vi "Target Gallon Fill Time.vi"(7 "Target Gallons":dbl, 8 "Error In":errorcluster, 9 "GEA Inputs":T1 {"Destination" format="%.0x"; "Source" format="%.0x"}, 10 "Standalone?":bool, 11 "GEA2 Reference In":refnum<k24>) -> (0 "Error Out":errorcluster, 2 "Target Gallon Fill Time (sec)":dbl, 3 "GEA2 Reference Out":refnum<k24>)   [LabVIEW 2016, in "TLMB.lvlib"]
uses:
  Projects/TLMB.lvlib
  Q:/Common/DLLs/GEA3/GeaCommunication.dll
  Common/DLLs/GEA3/GeaCommunication.dll
  Common/LabVIEW GEA2 Toolkit/LabVIEW_GEA2_Toolkit.lvlibp/type defs/Source_Destination.ctl
  Common/LabVIEW GEA2 Toolkit/LabVIEW_GEA2_Toolkit.lvlibp/type defs/ERD Read Data In.ctl
  Common/LabVIEW GEA2 Toolkit/LabVIEW_GEA2_Toolkit.lvlibp/type defs/Data Type.ctl
  Common/LabVIEW GEA2 Toolkit/LabVIEW_GEA2_Toolkit.lvlibp
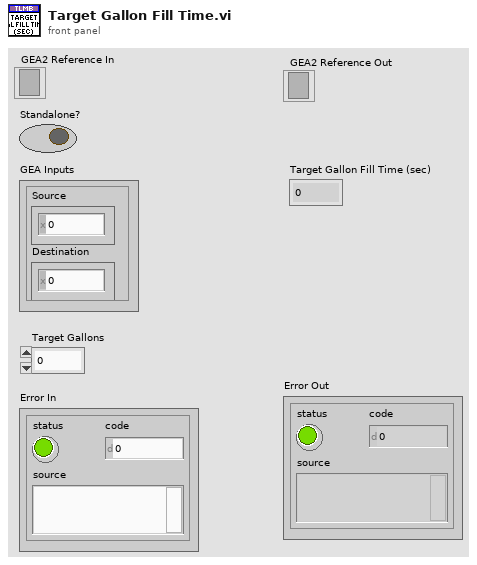
[diagram p1: front panel]
types:
  T1 = typedef "LabVIEW_GEA2_Toolkit.lvlibp/Source_Destination.ctl" = cluster{"Source":u8, "Destination":u8}
  T2 = typedef "LabVIEW_GEA2_Toolkit.lvlibp/ERD Read Data In.ctl" = cluster{"ERD Number":u16, "Data Type":T3}
  T3 = typedef "LabVIEW_GEA2_Toolkit.lvlibp/Data Type.ctl" = enum16{"string", "boolean", "uint8_t", "uint16_t", "uint32_t", "uint64_t", "int8_t", "int16_t", "int32_t", "int64_t"}
  T4 = typedef "LabVIEW_GEA2_Toolkit.lvlibp/ERD Read Data Out.ctl" = cluster{"ERD Number":u16, "Data":string}
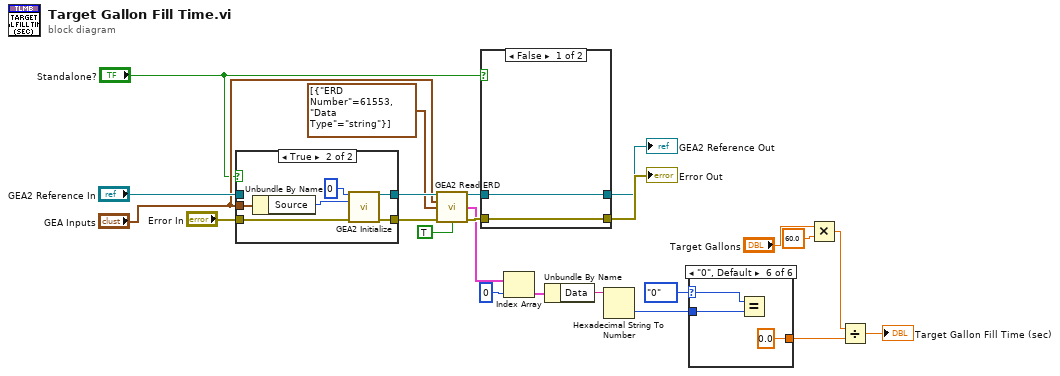
[diagram p0: block diagram]
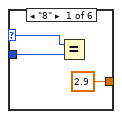
[diagram p2: hidden frame]
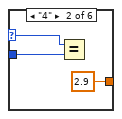
[diagram p3: hidden frame]
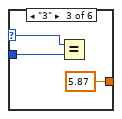
[diagram p4: hidden frame]
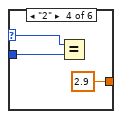
[diagram p5: hidden frame]
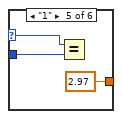
[diagram p6: hidden frame]
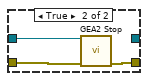
[diagram p7: hidden frame]
diagram:
  n1 = case shown="True" "Standalone?" {
    tunnel: "Error In" -> [w24 w31]
    tunnel: [w24 w30] -> w23
    tunnel: "GEA2 Reference In" -> [w25 _]
    tunnel: [w25 w29] -> w18
    tunnel: "GEA Inputs" -> [_ w27]
    frame False {
    }
    frame True {
      n2 = Unbundle By Name(w27) -> ("Source"=w28:u8)
      n3 = call "GEA2 Initialize.vi"("Board Index"=0, "Source Address"=w28, "error in"=w31) -> ("GEA2 Reference Out"=w29:refnum<k24>, "error out"=w30:errorcluster)  [unwired: 10 in, 1 out]
    }
  }
  n4 = call "GEA2 Read ERD.vi"("GEA2 Reference In"=w18, "GEA Inputs"="GEA Inputs", "Read ERD List"=T2[] [{"ERD Number"=61553, "Data Type"=enum."string"}], "Error In"=w23, "Verify ERD Response?"=TRUE) -> ("GEA2 Reference Out"=w16:refnum<k24>, "ERD Data Out"=w11:T4[], "Error Out"=w15:errorcluster)  [unwired: 7 in, 1 out]
  n5 = case shown="False" "Standalone?" {
    tunnel: w15 -> [w32 w36]
    tunnel: [w32 w35] -> w21
    tunnel: w16 -> [w33 w34]
    tunnel: [w33 _] -> w19
    frame False {
    }
    frame True {
      n6 = call "GEA2 Stop.vi"("GEA2 Reference In"=w34, "Error In"=w36) -> ("Error Out"=w35:errorcluster)  [unwired: 13 in]
    }
  }
  "Error Out" <- w21
  "GEA2 Reference Out" <- w19
  n7 = Index Array(array=w11, index=0) -> (element=w10:T4)
  n8 = Unbundle By Name(w10) -> ("Data"=w6:string)
  n9 = Hexadecimal String To Number(string=w6) -> (number=w5:u32)  [unwired: 2 in, 1 out]
  n10 = case shown="\"0\", Default" enum32{"8", "4", "3", "2", "1", "0"}."0" {
    selector: enum32{"8", "4", "3", "2", "1", "0"}."0" -> [w39 w42 w45 w48 w51 w53]
    tunnel: w5 -> [w38 w41 w44 w47 w50 w52]
    tunnel: [2.9 2.9 5.87 2.9 2.97 0.0] -> w4
    frame "8" {
      n11 = Equal?(x=w39, y=w38) -> ()  [unwired: 1 out]
    }
    frame "4" {
      n12 = Equal?(x=w42, y=w41) -> ()  [unwired: 1 out]
    }
    frame "3" {
      n13 = Equal?(x=w45, y=w44) -> ()  [unwired: 1 out]
    }
    frame "2" {
      n14 = Equal?(x=w48, y=w47) -> ()  [unwired: 1 out]
    }
    frame "1" {
      n15 = Equal?(x=w51, y=w50) -> ()  [unwired: 1 out]
    }
    frame "0", Default {
      n16 = Equal?(x=w53, y=w52) -> ()  [unwired: 1 out]
    }
  }
  n17 = Multiply(x="Target Gallons", y=60.0) -> (x*y=w8:dbl)
  n18 = Divide(x=w8, y=w4) -> (x/y=→"Target Gallon Fill Time (sec)":dbl)
